vi "IMAQController.InitPanel.vi"(0 "i ref in":refnum<vi>, 5 "error in":errorcluster) -> (14 "i ref out":refnum<vi>, 16 "Camera Config Array":string[][](array[string]), 17 "actCameras":i32[](array[numeric]), 19 "error out":errorcluster)   [LabVIEW 2014, in "IMAQController.lvlib"]
uses:
  IMAQController.lvlib
  CSCore/CSSystem/CoreLib/CoreLib.int 2 byte array.vi
  CSCore/CSSystem/CoreLib/CoreLib.byte array 2 string.vi
  CSCore/BaseProcess/BaseProcess.lvlib
  CSCore/CSSystem/CoreLib/CoreLib.lvlib
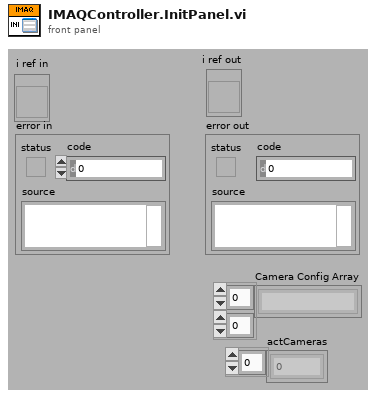
[diagram p1: front panel]
types:
  T1 = cluster{"Camera Name-Array":string[], "own Camera Type":string}
  T2 = typedef "IMAQController.lvlib/IMAQController.i attribute.ctl" = cluster{"ImageTakenID":i32, "actSequencer":string, "actScanner":string, "CameraTriggerID":i32, "activatedCameras":cluster{"Name":string, "Camera Type":string, "Acquisition Mode":u32, "JPEG Mode?":bool, "Acquisition Delay":dbl, "Save Images?":bool, "Center Coordinates":T3, "PixelPermm":cluster{"Horizontal":dbl, "Vertical":dbl}, "Rotation":dbl, "Mirror Mode":u32, "PixelCoordinates":cluster{"1":cluster{"Horizontal":i32, "Vertical":i32}, "2":cluster{"Horizontal":i32, "Vertical":i32}, "3":cluster{"Horizontal":i32, "Vertical":i32}, "4":cluster{"Horizontal":i32, "Vertical":i32}}, "RWCoordinates":cluster{"1":cluster{"Horizontal":dbl, "Vertical":dbl}, "2":cluster{"Horizontal":dbl, "Vertical":dbl}, "3":cluster{"Horizontal":dbl, "Vertical":dbl}, "4":cluster{"Horizontal":dbl, "Vertical":dbl}}, "HorizScaling":dbl, "VertScaling":dbl}[], "Ini C-Array":string[], "actCamera":string, "activeCamera":cluster{"Name":string, "Camera Type":string, "Aqcuisation Mode":enum32{"Internal Trigger", "Scan", "free Running", "External Trigger"}, "JPEG Mode?":bool, "Acquisition Delay":dbl, "Save Images?":bool, "Center Coordinates":T3, "PixelPermm":cluster{"Horizontal":dbl, "Vertical":dbl}, "Rotation":dbl, "Mirror Mode":u32, "PixelCoordinates":cluster{"1":cluster{"Horizontal":i32, "Vertical":i32}, "2":cluster{"Horizontal":i32, "Vertical":i32}, "3":cluster{"Horizontal":i32, "Vertical":i32}, "4":cluster{"Horizontal":i32, "Vertical":i32}}, "RWCoordinates":cluster{"1":cluster{"Horizontal":dbl, "Vertical":dbl}, "2":cluster{"Horizontal":dbl, "Vertical":dbl}, "3":cluster{"Horizontal":dbl, "Vertical":dbl}, "4":cluster{"Horizontal":dbl, "Vertical":dbl}}, "HorizScaling":dbl, "VertScaling":dbl}, "BilderMittelungen":u8, "OldPicture":dbl[][]}
  T3 = typedef "LVPoint32TypeDef.ctl" = cluster{"Horizontal":i32, "Vertical":i32}
  T4 = cluster{"Name":string, "Camera Type":string, "Acquisition Mode":u32, "JPEG Mode?":bool, "Acquisition Delay":dbl, "Save Images?":bool, "Center Coordinates":T3, "PixelPermm":cluster{"Horizontal":dbl, "Vertical":dbl}, "Rotation":dbl, "Mirror Mode":u32, "PixelCoordinates":cluster{"1":cluster{"Horizontal":i32, "Vertical":i32}, "2":cluster{"Horizontal":i32, "Vertical":i32}, "3":cluster{"Horizontal":i32, "Vertical":i32}, "4":cluster{"Horizontal":i32, "Vertical":i32}}, "RWCoordinates":cluster{"1":cluster{"Horizontal":dbl, "Vertical":dbl}, "2":cluster{"Horizontal":dbl, "Vertical":dbl}, "3":cluster{"Horizontal":dbl, "Vertical":dbl}, "4":cluster{"Horizontal":dbl, "Vertical":dbl}}, "HorizScaling":dbl, "VertScaling":dbl}[]
  T5 = cluster{"Name":string, "Camera Type":string, "Acquisition Mode":u32, "JPEG Mode?":bool, "Acquisition Delay":dbl, "Save Images?":bool, "Center Coordinates":T3, "PixelPermm":cluster{"Horizontal":dbl, "Vertical":dbl}, "Rotation":dbl, "Mirror Mode":u32, "PixelCoordinates":cluster{"1":cluster{"Horizontal":i32, "Vertical":i32}, "2":cluster{"Horizontal":i32, "Vertical":i32}, "3":cluster{"Horizontal":i32, "Vertical":i32}, "4":cluster{"Horizontal":i32, "Vertical":i32}}, "RWCoordinates":cluster{"1":cluster{"Horizontal":dbl, "Vertical":dbl}, "2":cluster{"Horizontal":dbl, "Vertical":dbl}, "3":cluster{"Horizontal":dbl, "Vertical":dbl}, "4":cluster{"Horizontal":dbl, "Vertical":dbl}}, "HorizScaling":dbl, "VertScaling":dbl}
  T6 = typedef "CoreDefs.call_type.ctl" = cluster{"Object":string, "Selector":string, "CallType":enum16{"simple", "synchronous", "asynchronous"}, "Async Object":string, "Async Selector":string, "Data Descriptor":T7, "Data":T8, "Error #":i32, "Expire":u32}
  T7 = typedef "BaseProcess.lvlib/BaseProcess.descriptor string definition.ctl" = string
  T8 = typedef "CoreDefs.rawDataType.ctl" = i8[]
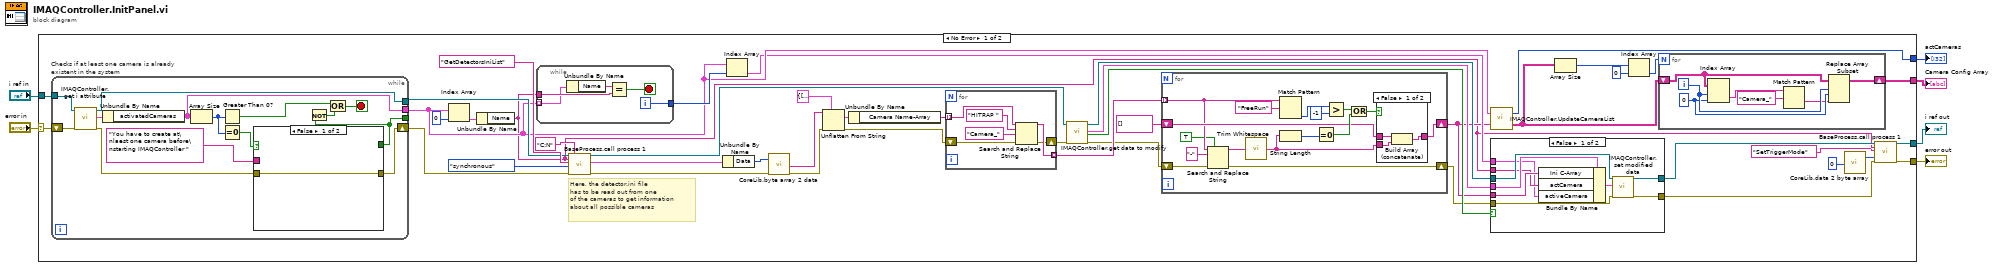
[diagram p0: block diagram]
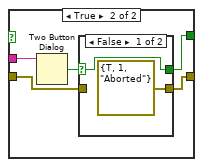
[diagram p4: hidden frame]
diagram:
  n1 = case shown="No Error" "error in" {
    selector: "error in" -> [w36 w126]
    tunnel: "i ref in" -> [w38 w125]
    tunnel: [w13 w126] -> w5
    tunnel: [w24 _] -> w4
    tunnel: [w11 w125] -> w2
    tunnel: [w28 _] -> w1
    frame No Error {
      # "Here, the detector.ini file\nhas to be read out from one\nof the cameras to get information\nabout all possible cameras"
      n2 = while "Checks if at least one camera is already existent in the system" {
        shift-right: [w106] -> w43
        shift-left: w36 -> [w114]
        tunnel: [w113] -> w42
        tunnel: [w111] -> w26
        tunnel: [w101] -> _
        tunnel: w38 -> [w105]
        stop <- w104 stop-if-true
        n3 = call "IMAQController.get i attribute.vi"("i ref in"=w105, "error in (no error)"=w114) -> ("i ref out"=w113:refnum<vi>, "i attribute"=w112:T2, "error out"=w107:errorcluster)  [unwired: 15 in]
        n4 = Unbundle By Name(w112) -> ("activatedCameras"=w111:T4)
        n5 = Array Size(array=w111) -> (size(s)=w109:i32)
        n6 = Greater Than 0?(x=w109) -> (x > 0?=w103:bool)
        n7 = Equal To 0?(x=w109) -> (x = 0?=w110:bool)
        n8 = case shown="False" w110 {
          tunnel: [_ w118] -> w101
          tunnel: "You have to create at\nlaest one camera before\nstarting IMAQController " -> [_ w120]
          tunnel: w107 -> [w115 w117]
          tunnel: [w115 w116] -> w106
          frame False {
          }
          frame True {
            n9 = Two Button Dialog(message=w120) -> (T button?=w119:bool)  [unwired: 2 in]
            n10 = case shown="False" w119 {
              selector: w119 -> [w122 w124]
              tunnel: [w122 w124] -> w118
              tunnel: w117 -> [_ w123]
              tunnel: [errorcluster {"status"=TRUE, "code"=1, "source"="Aborted"} ("error out") w123] -> w116
              frame False {
              }
              frame True {
              }
            }
          }
        }
        n11 = Not(x=w101) -> (.not. x?=w102:bool)
        n12 = Or(x=w103, y=w102) -> (x .or. y?=w104:bool)
      }
      n13 = Index Array(array=w26, index=0) -> (element=w50:T5)
      n14 = Unbundle By Name(w50) -> ("Name"=w10:string)
      n15 = while {
        tunnel: w26 -> [w82] mode=indexing
        tunnel: w10 -> [w83]
        tunnel: [w79] -> w27
        i -> [w79]
        stop <- w80 stop-if-true
        n16 = Unbundle By Name(w82) -> ("Name"=w81:string)
        n17 = Equal?(x=w81, y=w83) -> (x = y?=w80:bool)
      }
      n18 = call "BaseProcess.call process 1.vi"("i ref in"=w42, "Object"=w10, "Selector"="GetDetectorsIniList", "CallType"=enum16{"simple", "synchronous", "asynchronous"}."synchronous", "error in (no error)"=w43, "Data Descriptor"="C:N") -> ("i ref out"=w35:refnum<vi>, "call cluster out"=w47:T6, "error out"=w41:errorcluster)  [unwired: 11 in]
      n19 = Unbundle By Name(w47) -> ("Data"=w46:T8)
      n20 = Index Array(array=w26, index=w27) -> (element=w25:T5)
      n21 = call-poly "CoreLib.byte array 2 data.vi"("byteArray"=w46, "error in (no error)"=w41) -> ("string"=w45:string, "error out"=w40:errorcluster)  [unwired: 15 in, 1 out]
      n22 = Unflatten From String(type=T1 {"Camera Name-Array"=[], "own Camera Type"=""} ("CameraInfos"), binary string=w45, error in (no error)=w40) -> (value=w44:T1, error out=w30:errorcluster)  [unwired: 2 in, 1 out]
      n23 = Unbundle By Name(w44) -> ("Camera Name-Array"=w31:string[])
      n24 = for {
        tunnel: w31 -> [w89] mode=indexing
        tunnel: [w88] -> w19 mode=indexing
        shift-right: [w84] -> w29
        shift-left: w30 -> [w85]
        n25 = Search and Replace String(input string=w89, search string="HITRAP ", replace string="Camera_" ("replace string (\"\")"), error in=w85) -> (result string=w88:string, error out=w84:errorcluster)  [unwired: 4 in, 2 out]
      }
      n26 = call "IMAQController.get data to modify.vi"("i ref in"=w35, "error in (no error)"=w29) -> ("i ref out"=w33:refnum<vi>, "i attribute"=w32:T2, "timed out"=w34:bool, "error out"=w16:errorcluster)  [unwired: 14 in]
      n27 = for {
        tunnel: w19 -> [w57] mode=indexing
        shift-right: [w59] -> w17
        shift-left: string[] [] -> [w60]
        shift-right: [w52] -> w15
        shift-left: w16 -> [w53]
        n28 = Search and Replace String(replace all?=TRUE ("replace all? (F)"), input string=w57, search string="-", error in=w53) -> (result string=w55:string, error out=w52:errorcluster)  [unwired: 4 in, 2 out]
        n29 = call <vilib>:"Trim Whitespace.vi"("string"=w55) -> ("trimmed string"=w58:string)  [unwired: 1 in]
        n30 = Match Pattern(string=w57, regular expression="FreeRun") -> (offset past match=w65:i32)  [unwired: 1 in, 3 out]
        n31 = String Length(string=w58) -> (length=w67:i32)
        n32 = Equal To 0?(x=w67) -> (x = 0?=w61:bool)
        n33 = Greater?(x=w65, y=-1) -> (0:w62:bool)
        n34 = Or(x=w62, y=w61) -> (x .or. y?=w63:bool)
        n35 = case shown="False" w63 {
          tunnel: w60 -> [w70 w71]
          tunnel: [w69 w71] -> w59
          tunnel: w58 -> [w68 _]
          frame False {
            n36 = Build Array (concatenate)(w70, w68) -> (w69:string[])
          }
          frame True {
          }
        }
      }
      n37 = call "IMAQController.UpdateCameraList.vi"("activatedCameras"=w26, "Detector.ini List Camera-Array"=w17) -> ("actItem Number"=w28:i32[], "Item Names"=w23:string[][])  [unwired: 16 in]
      n38 = case shown="False" w34 {
        tunnel: w15 -> [w98 w100]
        tunnel: w33 -> [w96 w99]
        tunnel: [w97 w100] -> w14
        tunnel: [w95 w99] -> w12
        tunnel: w32 -> [w93 _]
        tunnel: w17 -> [w92 _]
        tunnel: w10 -> [w91 _]
        tunnel: w25 -> [w90 _]
        frame False {
          n39 = Bundle By Name(cluster=w93, "Ini C-Array"=w92, "actCamera"=w91, "activeCamera"=w90) -> (w94:T2)
          n40 = call "IMAQController.set modified data.vi"("i ref in"=w96, "i attribute"=w94, "error in (no error)"=w98) -> ("i ref out"=w95:refnum<vi>, "error out"=w97:errorcluster)  [unwired: 15 in]
        }
        frame True {
        }
      }
      n41 = Array Size(array=w23) -> (size(s)=w22:i32[])
      n42 = Index Array(array=w22, index=0) -> (element=w21:i32)
      n43 = for {
        N: w21 -> [_]
        shift-right: [w72] -> w24
        shift-left: w23 -> [w76]
        i -> [w75]
        w74 = 0 ("disabled index (col)")
        n44 = Index Array(array=w76, index (row)=w75, index (col)=w74) -> (element=w78:string)
        n45 = Match Pattern(string=w78, regular expression="Camera_") -> (after substring=w73:string)  [unwired: 1 in, 3 out]
        n46 = Replace Array Subset(array=w76, new element=w73, index (row)=w75, index (col)=w74) -> (w72:string[][])
      }
      n47 = call-poly "CoreLib.data 2 byte array.vi"("i32"=0) -> ("byteArray out"=w8:T8)  [unwired: 18 in]
      n48 = call "BaseProcess.call process 1.vi"("i ref in"=w12, "Object"=w10, "Selector"="SetTriggerMode", "Data"=w8, "error in (no error)"=w14) -> ("i ref out"=w11:refnum<vi>, "error out"=w13:errorcluster)  [unwired: 12 in, 1 out]
    }
    frame Error {
    }
  }
  "error out" <- w5
  "Camera Config Array" <- w4
  "i ref out" <- w2
  "actCameras" <- w1
